vi "Binary_SpectroscopyFile-ReadData.vi"(7 "Read Parameters only? (F)":bool, 8 "error in":errorcluster, 9 "Config":T1, 10 "Experiment to read (Index)":i32, 11 "File ref In":refnum<file>) -> (0 "error out":errorcluster, 1 "data":sgl[][](array[numeric]) format="%#_4p", 2 "Parameter values":sgl[](array[numeric]) format="%#_6p", 3 "File ref Out":refnum<file>)   [LabVIEW 2019, in "Nanonis Prog Interface.lvlib"]
doc: "<B>Reads spectroscopy data of the specified experiment (index).</B> \n\nIt returns the parameters (scalar values) like Z position as well as the spectroscopy channels (each row corresponds to a channel)."
uses:
  <userlib>/Nanonis Prog Interface V5/Nanonis Prog Interface.lvlib
  <userlib>/Nanonis Prog Interface V5/File/Binary_SpectroscopyFile-Config.ctl
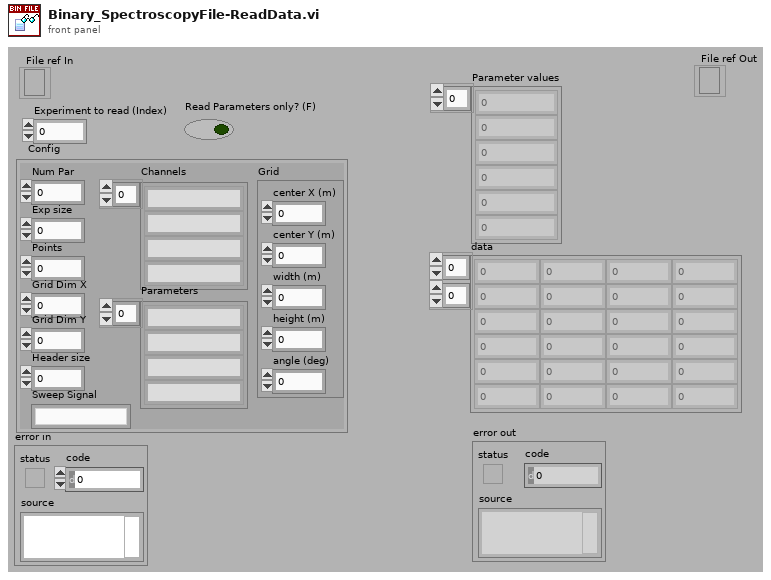
[diagram p1: front panel]
types:
  T1 = typedef "Nanonis Prog Interface.lvlib/Binary_SpectroscopyFile-Config.ctl" = cluster{"Num Par":i32, "Exp size":i32, "Points":i32, "Grid Dim X":i32, "Grid Dim Y":i32, "Header size":i32, "Channels":string[], "Parameters":string[], "Sweep Signal":string, "Grid":cluster{"center X (m)":sgl, "center Y (m)":sgl, "width (m)":sgl, "height (m)":sgl, "angle (deg)":sgl}}
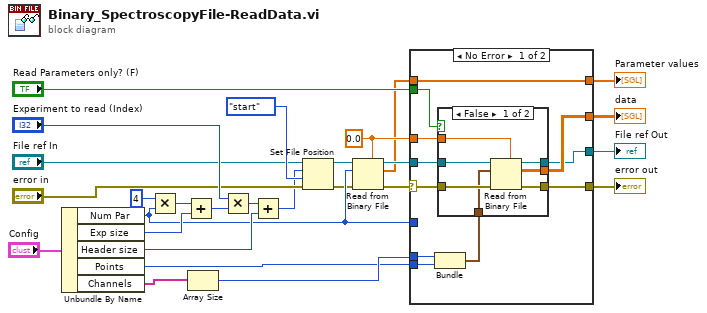
[diagram p0: block diagram]
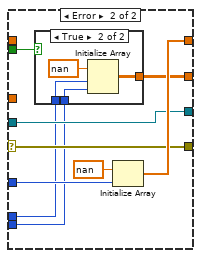
[diagram p3: hidden frame]
diagram:
  w22 = sgl 0.0
  n1 = Unbundle By Name("Config") -> ("Num Par"=w6:i32, "Exp size"=w13:i32, "Header size"=w10:i32, "Points"=w4:i32, "Channels"=w21:string[])
  n2 = Multiply(x=4, y=w6) -> (x*y=w26:i32)
  n3 = Add(x=w26, y=w13) -> (x+y=w24:i32)
  n4 = Array Size(array=w21) -> (size(s)=w5:i32)
  n5 = Multiply(x="Experiment to read (Index)", y=w24) -> (x*y=w12:i32)
  n6 = Add(x=w12, y=w10) -> (x+y=w11:i32)
  n7 = Set File Position(offset (in bytes) (0)=w11, refnum="File ref In", from (0:start)=enum16{"start", "end", "current"}."start" ("pos mode (0:2)"), error in="error in") -> (refnum out=w3:refnum<file>, error out=w2:errorcluster)
  n8 = Read from Binary File(5:w22, 8:w2, 10:w6, 11:w3) -> (0:w9:errorcluster, 2:w8:sgl[], 3:w23:refnum<file>)  [unwired: 2 in, 1 out]
  n9 = case shown="No Error" w9 {
    selector: w9 -> [w32 w53]
    tunnel: w23 -> [w38 w52]
    tunnel: w22 -> [w37 _]
    tunnel: [w36 w48] -> w20
    tunnel: [w35 w52] -> w19
    tunnel: [w34 w53] -> w16
    tunnel: "Read Parameters only? (F)" -> [w33 w51]
    tunnel: w8 -> [w31 _]
    tunnel: [w31 w54] -> w7
    tunnel: w6 -> [_ w56]
    tunnel: w5 -> [w30 w50]
    tunnel: w4 -> [w29 w49]
    frame No Error {
      n10 = Bundle(w30, "Points"=w29) -> (w28:cluster{i32, "Points":i32})  [unwired: 1 in]
      n11 = case shown="False" w33 {
        tunnel: w38 -> [w45 w47]
        tunnel: w32 -> [w44 w46]
        tunnel: w28 -> [w43 _]
        tunnel: w37 -> [w42 _]
        tunnel: [w41 _] -> w36
        tunnel: [w40 w47] -> w35
        tunnel: [w39 w46] -> w34
        frame False {
          n12 = Read from Binary File(5:w42, 8:w44, 10:w43, 11:w45) -> (0:w39:errorcluster, 2:w41:sgl[][], 3:w40:refnum<file>)  [unwired: 2 in, 1 out]
        }
        frame True {
        }
      }
    }
    frame Error {
      n13 = case shown="True" w51 {
        tunnel: w50 -> [_ w59]
        tunnel: w49 -> [_ w58]
        tunnel: [_ w57] -> w48
        frame False {
        }
        frame True {
          n14 = Initialize Array(sgl nan ("element"), w59, w58) -> (w57:sgl[][])
        }
      }
      n15 = Initialize Array(sgl nan ("element"), w56) -> (w54:sgl[])
    }
  }
  "Parameter values" <- w7
  "data" <- w20
  "error out" <- w16
  "File ref Out" <- w19
